vi "Proiect Rn Toth David-Andrei 633 AB-Detectarea defectiunilor pieselor auto.vi"() -> ()   [LabVIEW 2024]
uses:
  <vilib>/vision/NI_Vision_Development_Module.lvlib
panel:
  out "Status piesa":string
  in  "error in (no error) 2":errorcluster
  out "error out 2":errorcluster
  in  "Butonul de oprire":bool
  out "error out":errorcluster
  in  "error in (no error)":errorcluster
  in  "Calea imaginii care urmeaza sa fie verificata":path
  out "Imaginea finala":T1(plugin-control)
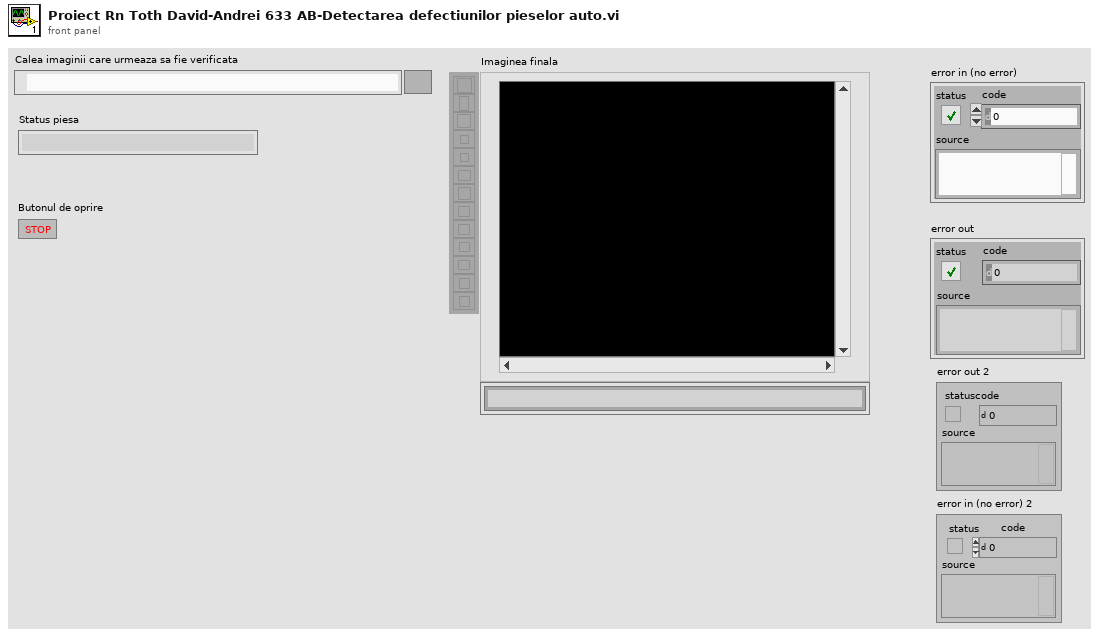
[diagram p1: front panel]
types:
  T1 = typedef "IMAQ Image.ctl" = refnum<image>
  T2 = enum32{"AutoM", "Close", "Dilate", "Erode", "Gradient", "Gradient out", "Gradient in", "Hit miss", "Open", "PClose", "POpen", "Thick", "Thin"}
  T3 = typedef "Image Type" = u32
  T4 = cluster{"Area":dbl, "Number of Holes":dbl, "Bounding Rect":cluster{"Left":dbl, "Top":dbl, "Right":dbl, "Bottom":dbl}, "Center of Mass":cluster{"X":dbl, "Y":dbl}, "Orientation":dbl, "Dimensions":cluster{"Width":dbl, "Height":dbl}}[]
  T5 = cluster{"Left":dbl, "Top":dbl, "Right":dbl, "Bottom":dbl}
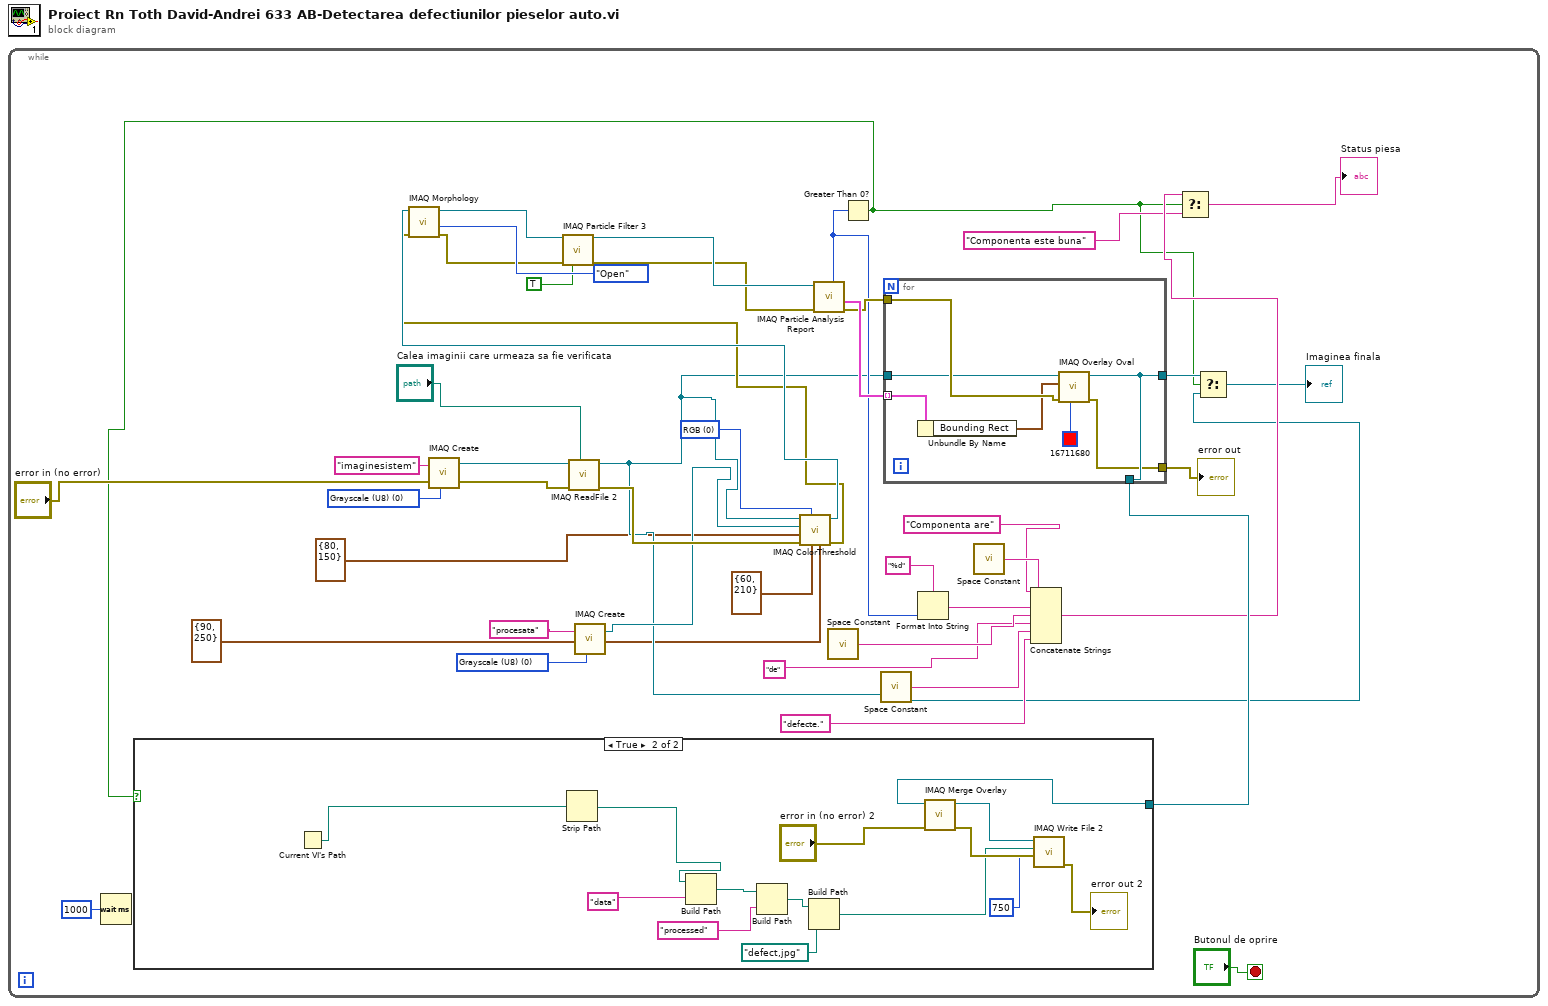
[diagram p0: block diagram]
diagram:
  n1 = while {
    stop <- "Butonul de oprire" stop-if-true
    w22 = u16 0 items=["RGB", "HSL", "HSV", "HSI"] ("Color Mode")
    w34 = T3 0 items=["Grayscale (U8)", "Grayscale (I16)", "Grayscale (SGL)", "Complex (CSG)", "RGB (U32)", "HSL (U32)", "RGB (U64)", "Grayscale (U16)"] ("Image Type")
    w43 = T3 0 items=["Grayscale (U8)", "Grayscale (I16)", "Grayscale (SGL)", "Complex (CSG)", "RGB (U32)", "HSL (U32)", "RGB (U64)", "Grayscale (U16)"] ("Image Type")
    n2 = Wait (ms)(milliseconds to wait=u32 1000) -> ()  [unwired: 1 out]
    n3 = call "IMAQ Create"("Image Name"="imaginesistem", "Image Type"=w43, "error in (no error)"="error in (no error)") -> ("New Image"=w41:T1, "error out"=w42:errorcluster)  [unwired: 2 in]
    n4 = call "IMAQ ReadFile 2"("File Path"="Calea imaginii care urmeaza sa fie verificata", "error in (no error)"=w42, "Image"=w41) -> ("error out"=w21:errorcluster, "Image Out"=w5:T1)  [unwired: 4 in, 3 out]
    n5 = call "IMAQ Create"("Image Name"="procesata", "Image Type"=w34) -> ("New Image"=w20:T1)  [unwired: 3 in, 1 out]
    n6 = call "IMAQ ColorThreshold"("Blue or Luma or Val or Inten Range"=cluster{"Lower value":i32, "Upper value":i32} {"Lower value"=90, "Upper value"=250}, "Green or Sat Range"=cluster{"Lower value":i32, "Upper value":i32} {"Lower value"=60, "Upper value"=210}, "Color Mode"=w22, "error in (no error)"=w21, "Red or Hue Range"=cluster{"Lower value":i32, "Upper value":i32} {"Lower value"=80, "Upper value"=150}, "Image Dst"=w20, "Image Src"=w5) -> ("error out"=w9:errorcluster, "Image Dst Out"=w11:T1)  [unwired: 3 in]
    n7 = call "IMAQ Morphology"("error in (no error)"=w9, "Operation"=T2."Open", "Image Src"=w11) -> ("error out"=w8:errorcluster, "Image Dst Out"=w13:T1)  [unwired: 7 in]
    n8 = call "IMAQ Particle Filter 3"("Image Src"=w13, "error in (no error)"=w8, "Reject Border? (F)"=TRUE) -> ("Image Dst Out"=w12:T1, "error out"=w10:errorcluster)  [unwired: 10 in, 1 out]
    n9 = call "IMAQ Particle Analysis Report"("error in (no error)"=w10, "Image"=w12) -> ("error out"=w37:errorcluster, "Particle Reports (Real-World)"=w39:T4, "Number of Particles"=w19:i32)  [unwired: 4 in, 3 out]
    n10 = call <vilib>:"Space Constant.vi"() -> ("String"=w27:string)
    n11 = Greater Than 0?(x=w19) -> (x > 0?=w4:bool)
    n12 = call <vilib>:"Space Constant.vi"() -> ("String"=w25:string)
    n13 = for {
      tunnel: w39 -> [w65] mode=indexing
      tunnel: [w61] -> w6
      tunnel: [w60] -> w38
      tunnel: w37 -> [w63]
      tunnel: w5 -> [w62]
      tunnel: [w61] -> w23
      n14 = Unbundle By Name(w65) -> ("Bounding Rect"=w59:T5)
      n15 = call "IMAQ Overlay Oval"("Color"=u32 16711680, "error in (no error)"=w63, "Bounding Rectangle"=w59, "Image"=w62) -> ("error out"=w60:errorcluster, "Image Out"=w61:T1)  [unwired: 6 in]
    }
    "error out" <- w38
    n16 = case shown="True" w4 {
      tunnel: w23 -> [_ w57]
      frame False {
      }
      frame True {
        n17 = Current VI's Path() -> (path=w52:path)
        n18 = Strip Path(path=w52) -> (stripped path=w51:path)  [unwired: 1 out]
        n19 = Build Path(base path=w51, name or relative path="data") -> (appended path=w49:path)
        n20 = Build Path(base path=w49, name or relative path="processed") -> (appended path=w47:path)
        n21 = Build Path(base path=w47, name or relative path=path "defect,jpg") -> (appended path=w46:path)
        n22 = call "IMAQ Merge Overlay"("error in (no error)"="error in (no error) 2", "Image Src"=w57) -> ("error out"=w58:errorcluster, "Image Dst Out"=w56:T1)  [unwired: 8 in]
        n23 = call-poly "IMAQ Write File 2"("error in (no error)"=w58, "Image Quality"=u32 750, "File Path"=w46, "Image"=w56) -> ("error out"=→"error out 2":errorcluster)  [unwired: 6 in, 1 out]
      }
    }
    n24 = Format Into String "Format Into String"(format string="%d", w19) -> (resulting string=w28:string)  [unwired: 2 in, 1 out]
    n25 = call <vilib>:"Space Constant.vi"() -> ("String"=w30:string)
    n26 = Concatenate Strings "Concatenate Strings"("Componenta are" ("string"), w30, w28, w27, "de", w25, "defecte." ("string")) -> (w17:string)
    n27 = Select(t=w17, s=w4, f="Componenta este buna") -> (s? t:f=→"Status piesa":string)
    n28 = Select(t=w6, s=w4, f=w5) -> (s? t:f=→"Imaginea finala":T1)
  }
